vi "allocate interface.vi"(11 "Slave Info List":T2(array[cluster])) -> ()   [LabVIEW 2013, in "dynamic profibus.lvlib"]
uses:
  dynamic profibus.lvlib
  data table allocation.ctl
panel:
  out "devices":T1[](array[typedef])
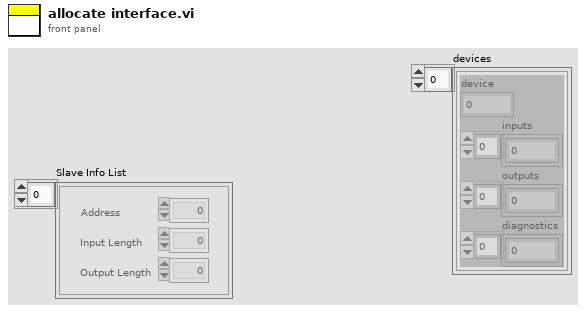
[diagram p1: front panel]
types:
  T1 = typedef "dynamic profibus.lvlib/data table allocation.ctl" = cluster{"device":i8, "inputs":u8[], "outputs":u8[], "diagnostics":u8[]}
  T2 = cluster{"Address":i8, "Input Length":u8, "Output Length":u8}[]
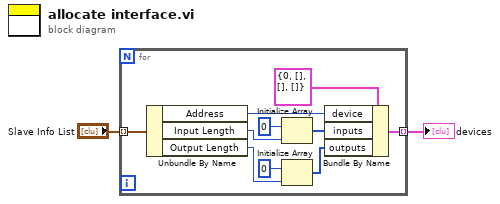
[diagram p0: block diagram]
diagram:
  n1 = for {
    tunnel: "Slave Info List" -> [w12] mode=indexing
    tunnel: [w3] -> w1 mode=indexing
    n2 = Unbundle By Name(w12) -> ("Address"=w4:i8, "Input Length"=w9:u8, "Output Length"=w7:u8)
    n3 = Initialize Array(u8 0, w9) -> (w5:u8[])
    n4 = Initialize Array(u8 0, w7) -> (w6:u8[])
    n5 = Bundle By Name(cluster=T1 {"device"=0, "inputs"=[], "outputs"=[], "diagnostics"=[]}, "device"=w4, "inputs"=w5, "outputs"=w6) -> (w3:T1)
  }
  "devices" <- w1
